vi "Adv_SetFullFrame.vi"(8 "error in (no error)":errorcluster, 11 "LightField Automation in":refnum<class "LightField Automation.lvclass">) -> (0 "error out":errorcluster, 3 "LightField Automation out":refnum<class "LightField Automation.lvclass">)   [LabVIEW 2019, in "LightField Automation.lvclass"]
uses:
  LightField Automation.lvclass
  C:/Program Files/Princeton Instruments/LightField/AddInViews/PrincetonInstruments.LightFieldViewV3.dll
  Program Files/Princeton Instruments/LightField/AddInViews/PrincetonInstruments.LightFieldViewV3.dll
  C:/Program Files/Princeton Instruments/LightField/PrincetonInstruments.LightFieldAddInSupportServices.dll
  Program Files/Princeton Instruments/LightField/PrincetonInstruments.LightFieldAddInSupportServices.dll
panel:
  in  "Heigth":i32=28
  in  "Width":i32=1340
  in  "X":i32
  in  "XBinning":i32=1
  in  "YBinning":i32=28
  in  "Y":i32=30
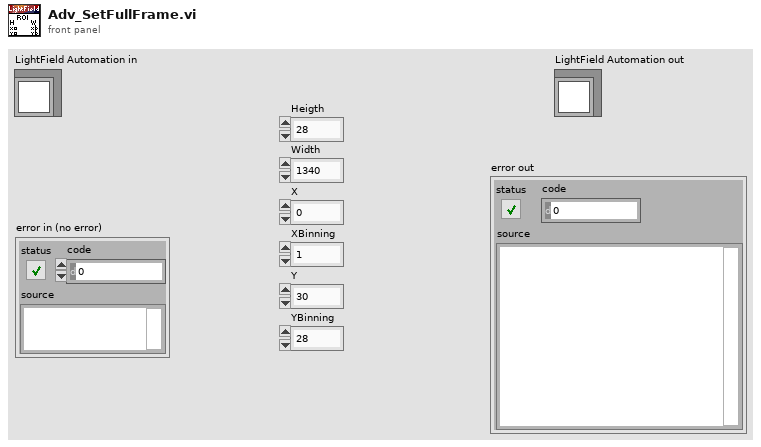
[diagram p1: front panel]
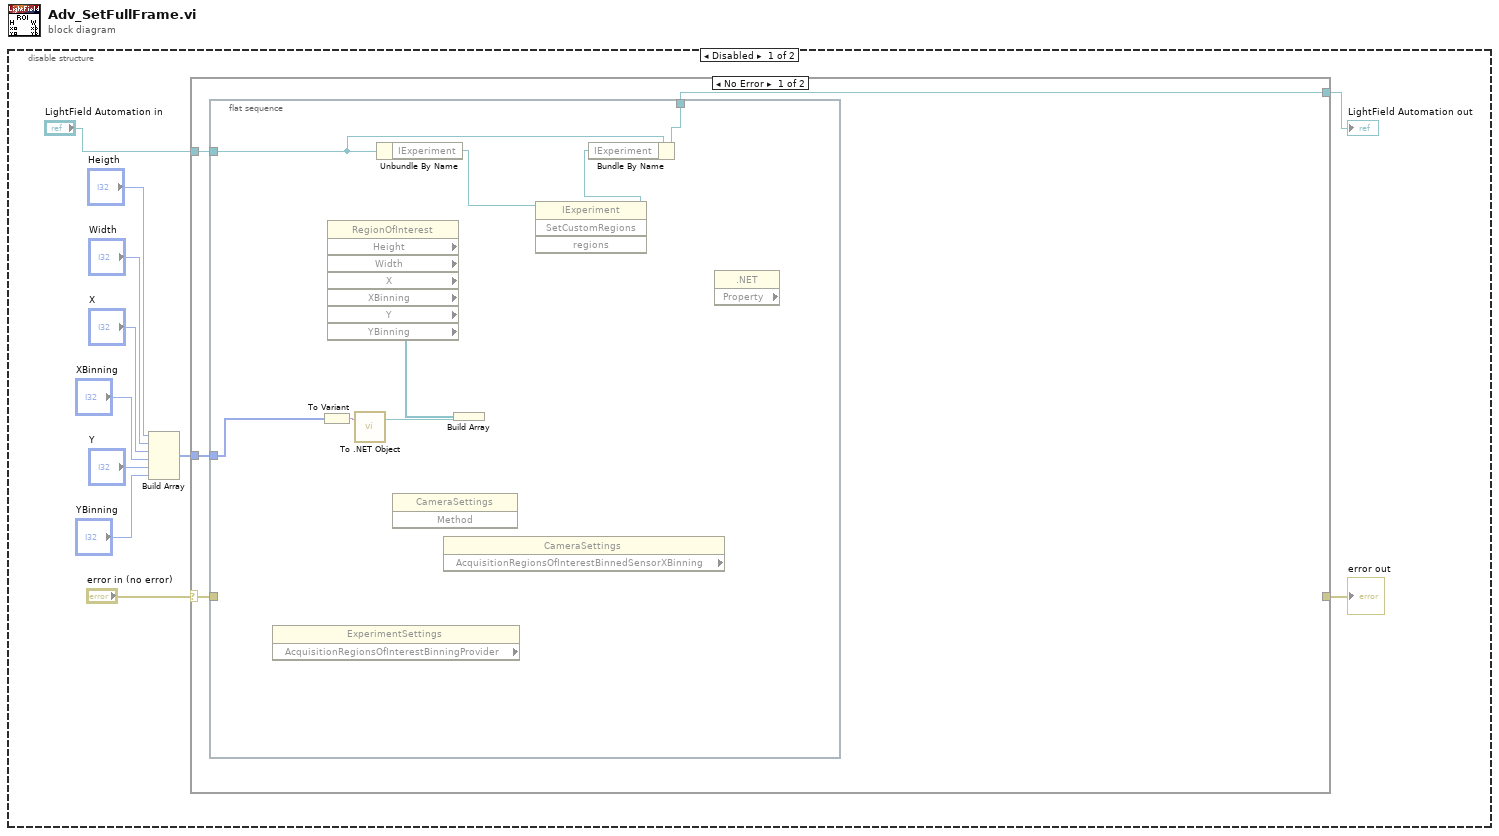
[diagram p0: block diagram]
diagram:
  n1 = disable-structure shown="Disabled" {
    frame Disabled {
      n2 = Build Array("Heigth", "Width", "X", "XBinning", "Y", "YBinning") -> (w4:i32[])
      n3 = case shown="No Error" "error in (no error)" {
        selector: "error in (no error)" -> [w15 w24]
        tunnel: [_ w24] -> w10
        tunnel: w4 -> [w14 _]
        tunnel: "LightField Automation in" -> [w13 _]
        tunnel: [w12 _] -> w1
        frame No Error {
          n4 = flat-sequence {
            tunnel: w15 -> [_]
            tunnel: w14 -> [w18]
            tunnel: w13 -> [w21]
            tunnel: [w20] -> w12
            frame #0 {
              n5 = property class="ExperimentSettings" props=["AcquisitionRegionsOfInterestBinningProvider"]() -> ()  [unwired: 2 in, 3 out]
              n6 = To Variant(anything=w18) -> (Variant=w19:variant)
              n7 = call <vilib>:"To .NET Object.vi"("anything"=w19) -> (".NET object"=w17:refnum<k24>)  [unwired: 1 in, 1 out]
              n8 = Unbundle By Name(w21) -> ("IExperiment"=w23:refnum<k24>)
              n9 = invoke class="CameraSettings" method=#-1() -> ()  [unwired: 3 in, 3 out]
              n10 = property class="CameraSettings" props=["AcquisitionRegionsOfInterestBinnedSensorXBinning"]() -> ()  [unwired: 2 in, 3 out]
              n11 = Build Array(w17) -> (w16:refnum<k24>[])
              n12 = property class="RegionOfInterest" props=["Height", "Width", "X", "XBinning", "Y", "YBinning"](reference=w16) -> ()  [unwired: 1 in, 8 out]
              n13 = invoke class="IExperiment" method="SetCustomRegions"(reference=w23) -> (reference out=w22:refnum<k24>)  [unwired: 3 in, 3 out]
              n14 = Bundle By Name(cluster=w21, "IExperiment"=w22) -> (w20:refnum<class "LightField Automation.lvclass">)
              n15 = property class=".NET" props=[]() -> ()  [unwired: 2 in, 3 out]
            }
          }
        }
        frame Error {
        }
      }
      "LightField Automation out" <- w1
      "error out" <- w10
    }
    frame Enabled {
    }
  }
